vi "Crea Dir For Decrypted.vi"(8 "error in (no error)":errorcluster, 11 "Crypter.lvclass":refnum<class "Crypter.lvclass">) -> (0 "error out":errorcluster, 2 "PathFolderForDecrypted":path, 3 "Crypter.lvclass 2":refnum<class "Crypter.lvclass">)   [LabVIEW 2016, in "Crypter.lvclass"]
uses:
  Crypter.lvclass
  Folder_Mgmt/Folder_Mgmt.lvclass
  Folder_Mgmt/Folder_Mgmt.lvclass/Folder_Mgmt.ctl
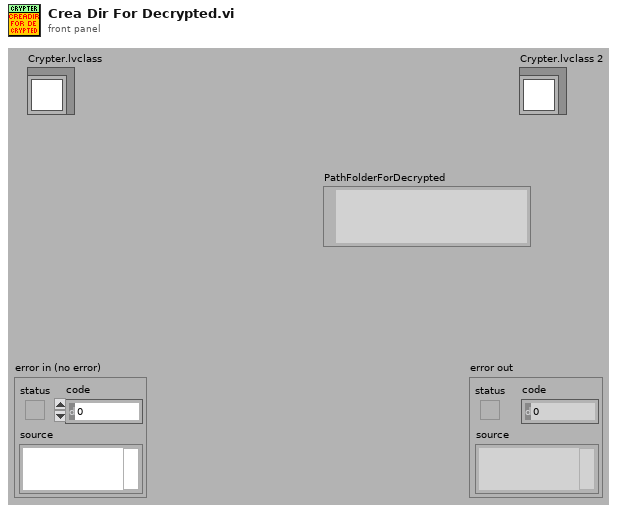
[diagram p1: front panel]
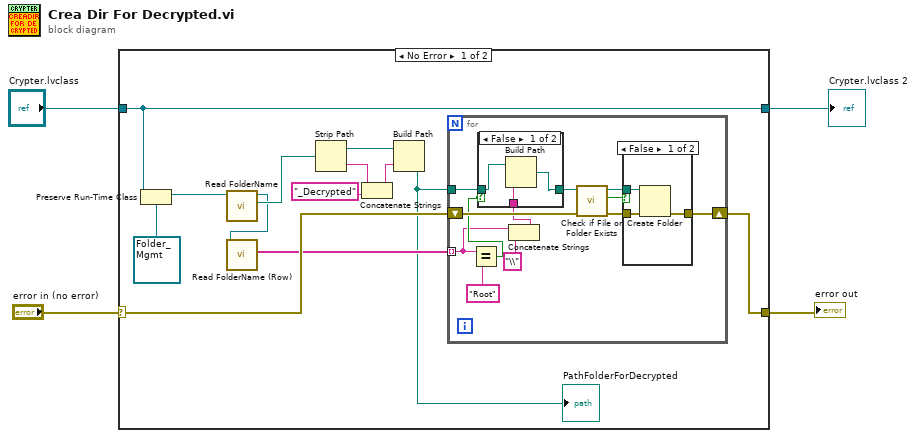
[diagram p0: block diagram]
diagram:
  n1 = case shown="No Error" "error in (no error)" {
    selector: "error in (no error)" -> [w13 w39]
    tunnel: [w12 w39] -> w3
    tunnel: [w10 w38] -> w1
    tunnel: "Crypter.lvclass" -> [w10 w38]
    frame No Error {
      n2 = Preserve Run-Time Class(object in=w10, 2:refnum<class "Folder_Mgmt.lvclass"> refnum ("Folder_Mgmt.lvclass")) -> (object out=w9:refnum<class "Folder_Mgmt.lvclass">)  [unwired: 1 in, 1 out]
      n3 = call "Read FolderName.vi"("Folder_Mgmt in"=w9) -> ("FolderName"=w8:path, "Folder_Mgmt out"=w7:refnum<class "Folder_Mgmt.lvclass">)  [unwired: 8 in, 1 out]
      n4 = call "Read FolderName (Row).vi"("Folder_Mgmt in"=w7) -> ("FolderName (Row)"=w6:string[])  [unwired: 8 in, 2 out]
      n5 = Strip Path(path=w8) -> (stripped path=w14:path, name=w16:string)
      n6 = Concatenate Strings(w16, "_Decrypted") -> (w15:string)
      n7 = Build Path(base path=w14, name or relative path=w15) -> (appended path=w5:path)
      "PathFolderForDecrypted" <- w5
      n8 = for {
        tunnel: w5 -> [w22]
        shift-right: [w25] -> w12
        shift-left: w13 -> [w26]
        tunnel: w6 -> [w20] mode=indexing
        n9 = Equal?(x=w20, y="Root") -> (x = y?=w23:bool)
        n10 = Concatenate Strings(w20, "\\" ("string")) -> (w18:string)
        n11 = case shown="False" w23 {
          tunnel: w22 -> [w32 w33]
          tunnel: [w30 w33] -> w21
          tunnel: w18 -> [w31 _]
          frame False {
            n12 = Build Path(base path=w32, name or relative path=w31) -> (appended path=w30:path)
          }
          frame True {
          }
        }
        n13 = call <vilib>:"Check if File or Folder Exists.vi"("error in (no error)"=w26, "path"=w21) -> ("error out"=w28:errorcluster, "file or folder exists?"=w29:bool, "dup path"=w27:path)  [unwired: 7 in]
        n14 = case shown="False" w29 {
          tunnel: w27 -> [w36 _]
          tunnel: w28 -> [w35 w37]
          tunnel: [w34 w37] -> w25
          frame False {
            n15 = Create Folder(path (use dialog)=w36, error in=w35) -> (error out=w34:errorcluster)  [unwired: 1 in, 2 out]
          }
          frame True {
          }
        }
      }
    }
    frame Error {
    }
  }
  "error out" <- w3
  "Crypter.lvclass 2" <- w1
